vi "Test.vi"() -> ()   [LabVIEW 2015]
uses:
  Queued Listbox.xctl
panel:
  in  "Selections":string[](array[string])=["asd", "ads"]
  out "Array - String":string[](array[string])=["asd", "ads"]
  out "error out":errorcluster
  in  "Strings":string[](array[string])=["s", "asd", "ads"]
  in  "Queued Listbox":string[](xcontrol)=["asd", "ads"]
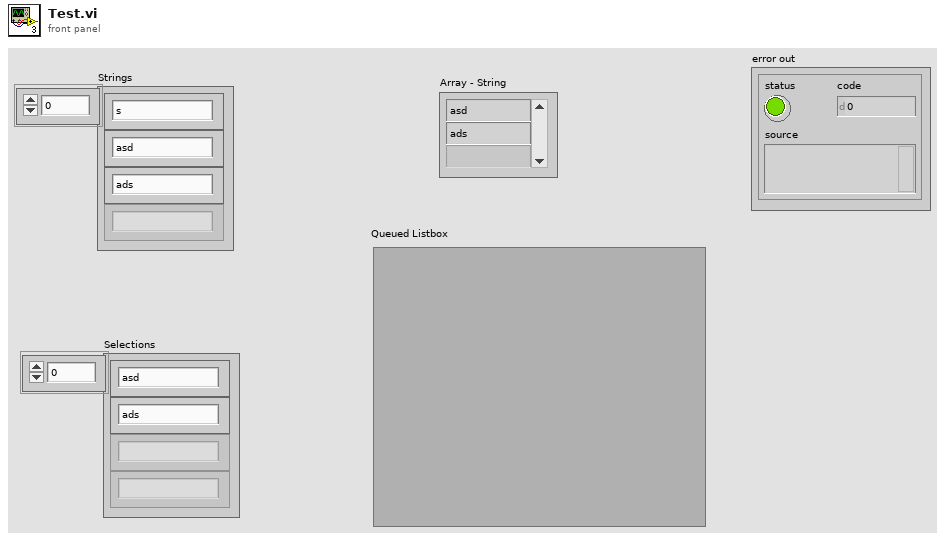
[diagram p1: front panel]
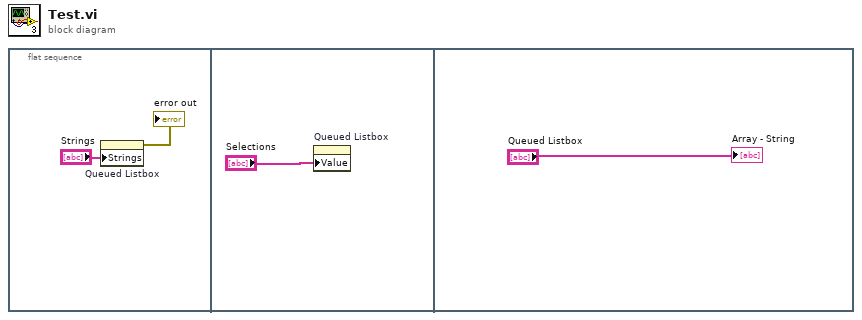
[diagram p0: block diagram]
diagram:
  n1 = flat-sequence {
    frame #0 {
      n2 = property on="Queued Listbox" class="Queued Listbox (strict)"("Strings"="Strings") -> (error out=→"error out":errorcluster)  [unwired: 2 in, 1 out]
    }
    frame #1 {
      n3 = property on="Queued Listbox" class="Queued Listbox (strict)"("Value"="Selections") -> ()  [unwired: 2 in, 2 out]
    }
    frame #2 {
      "Array - String" <- "Queued Listbox"
    }
  }
